vi "Close.vi"(8 "error in (no error)":errorcluster, 11 "APS 7050":refnum<class "APS 7050.lvclass">) -> (0 "error out":errorcluster, 3 "APS 7050 out":refnum<class "APS 7050.lvclass">)   [LabVIEW 2025, in "Power Supply.lvlib" / "APS 7050.lvclass"]
uses:
  APS 7050.lvclass
  APS 7050.lvclass/APS 7050.ctl
  <instrlib>/APS-7000 Series/APS-7000 Series.lvlib
  PS Instrument/Power Supply Instrument.lvclass
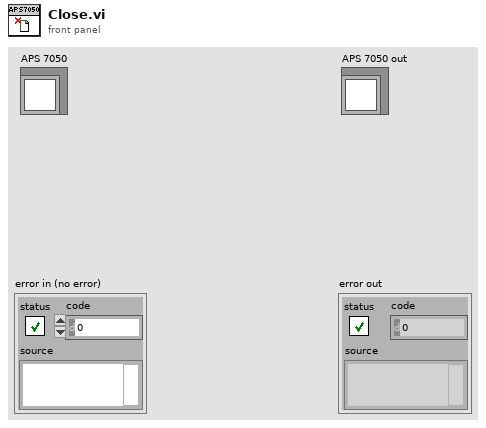
[diagram p1: front panel]
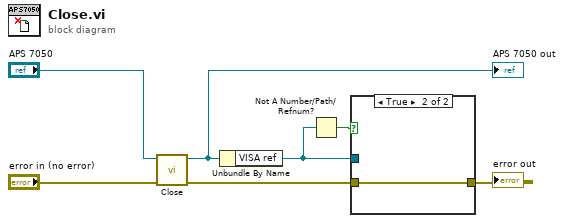
[diagram p0: block diagram]
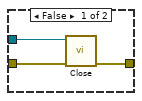
[diagram p2: hidden frame]
diagram:
  n1 = call-parent <instrlib>:"Close.vi"("error in (no error)"="error in (no error)", "Power Supply Instrument in"="APS 7050") -> ("error out"=w3:errorcluster, "Power Supply Instrument out"=w1:refnum<class "APS 7050.lvclass">)  [unwired: 8 in]
  "APS 7050 out" <- w1
  n2 = Unbundle By Name(w1) -> ("VISA ref"=w4:refnum<visa-resource-name>)
  n3 = Not A Number/Path/Refnum?(number/path/refnum=w4) -> (NaN/Path/Refnum?=w7:bool)
  n4 = case shown="True" w7 {
    tunnel: w3 -> [w9 w11]
    tunnel: [w10 w11] -> w6
    tunnel: w4 -> [w8 _]
    frame False {
      n5 = call <instrlib>:"Close.vi"("error in (no error)"=w9, "VISA resource name"=w8) -> ("error out"=w10:errorcluster)  [unwired: 9 in]
    }
    frame True {
    }
  }
  "error out" <- w6
